vi "Build Specifications.vi"(8 "Error In":errorcluster) -> (0 "Error Out":errorcluster, 3 "Build Specifications":string[](array[string]))   [LabVIEW 2017, in "Scripts.lvlib"]
uses:
  Scripts.lvlib
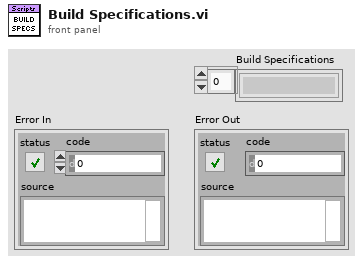
[diagram p1: front panel]
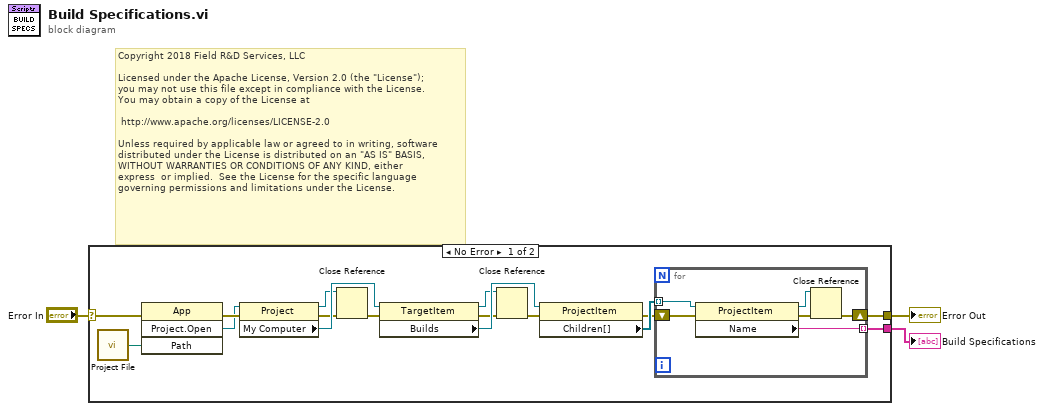
[diagram p0: block diagram]
diagram:
  # "Copyright 2018 Field R&D Services, LLC\n\nLicensed under the Apache License, Version 2.0 (the \"License\");\nyou may not use this file except in compliance with the License.\nYou may obtain a copy of the License at\n\n\thttp://www.apache.org/licenses/LICENSE-2.0\n\nUnless required by applicable law or agreed to in writing, software\ndistributed under the License is distributed on an \"AS IS\" BASIS,\nWITHOUT WARRANTIES OR CONDITIONS OF ANY KIND, either \nexpress  or implied.  See the License for the specific language \ngoverning permissions and limitations under the License."
  n1 = case shown="No Error" "Error In" {
    selector: "Error In" -> [w7 w26]
    tunnel: [w9 _] -> w3
    tunnel: [w8 w26] -> w2
    frame No Error {
      n2 = call "Project File.vi"() -> ("Project File"=w5:path)
      n3 = invoke class="App" method="Project.Open"(error in=w7, "Path"=w5) -> (error out=w6:errorcluster, "Project:Open"=w4:refnum<vi>)  [unwired: 2 in, 2 out]
      n4 = property class="Project"(reference=w4, error in=w6) -> (reference out=w16:refnum<vi>, error out=w17:errorcluster, "My Computer"=w19:refnum<vi>)
      n5 = Close Reference(reference=w16, error in (no error)=w17) -> (error out=w15:errorcluster)
      n6 = property class="TargetItem"(reference=w19, error in=w15) -> (reference out=w13:refnum<vi>, error out=w14:errorcluster, "Builds"=w18:refnum<vi>)
      n7 = Close Reference(reference=w13, error in (no error)=w14) -> (error out=w12:errorcluster)
      n8 = property class="ProjectItem"(reference=w18, error in=w12) -> (error out=w10:errorcluster, "Children[]"=w11:refnum<vi>[])  [unwired: 1 out]
      n9 = for {
        tunnel: w11 -> [w25] mode=indexing
        shift-right: [w21] -> w8
        shift-left: w10 -> [w24]
        tunnel: [w22] -> w9 mode=indexing
        n10 = property class="ProjectItem"(reference=w25, error in=w24) -> (reference out=w20:refnum<vi>, error out=w23:errorcluster, "Name"=w22:string)
        n11 = Close Reference(reference=w20, error in (no error)=w23) -> (error out=w21:errorcluster)
      }
    }
    frame Error {
    }
  }
  "Build Specifications" <- w3
  "Error Out" <- w2
